vi "Incrementer with registered output.vi"(4 "INC?":bool) -> (1 "count":u32)   [LabVIEW 2012]
doc: "This counter counts from 0....Rollover and then returns to zero\ne.g., If rollover is 2, counter moves as 0,1,2,0,1,2.....\n\n<Latency> = 1 Tick from Reset"
uses:
  <vilib>/rvi/FXPMathLib/basic elements/FxpDiscreteDelay/XNode/nifxpmath_DiscreteDelay.xnode
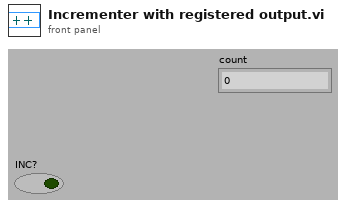
[diagram p1: front panel]
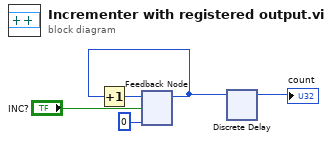
[diagram p0: block diagram]
diagram:
  n1 = feedback #1(u32 0) -> (w2:u32)
  n2 = Increment(x=w2) -> (x+1=w3:u32)
  n3 = feedback-in #1(w3, "INC?") -> ()
  n4 = xnode "Discrete Delay"("D"=w2) -> ("Q"=→"count":u32)
